vi "Read Timeout.vi"(8 "error in (no error)":errorcluster, 11 "Repeat Until Timeout in":refnum<class "bt_Repeat Until Timeout.lvclass">) -> (0 "error out":errorcluster, 2 "Timeout":dbl, 3 "Repeat Until Timeout out":refnum<class "bt_Repeat Until Timeout.lvclass">)   [LabVIEW 2021, in "BT.lvlib" / "bt_Repeat Until Timeout.lvclass"]
uses:
  bt_Repeat Until Timeout.lvclass
  bt_Repeat Until Timeout.lvclass/bt_Repeat Until Timeout.ctl
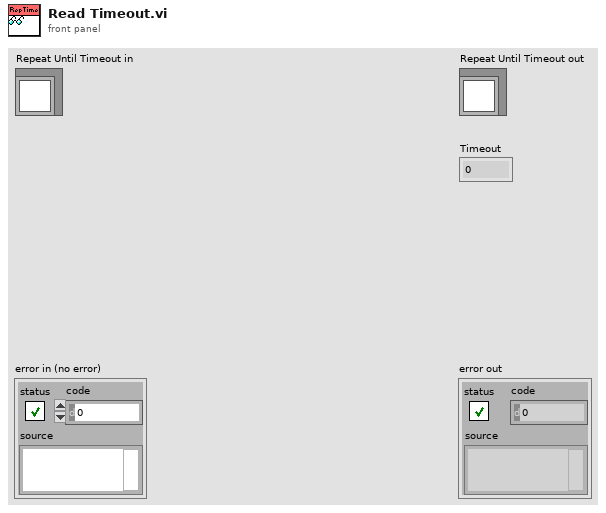
[diagram p1: front panel]
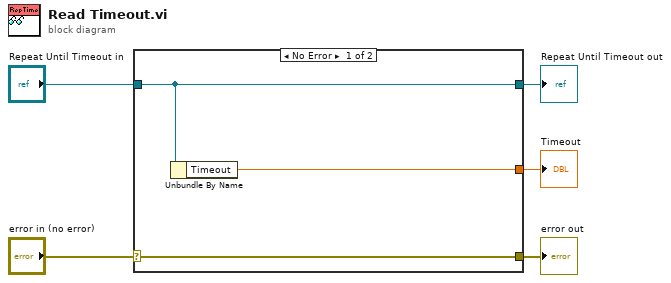
[diagram p0: block diagram]
diagram:
  n1 = case shown="No Error" "error in (no error)" {
    selector: "error in (no error)" -> [w8 w9]
    tunnel: [w8 w9] -> w4
    tunnel: [w7 w10] -> w2
    tunnel: "Repeat Until Timeout in" -> [w7 w10]
    tunnel: [w6 _] -> w1
    frame No Error {
      n2 = Unbundle By Name(w7) -> ("Timeout"=w6:dbl)
    }
    frame Error {
    }
  }
  "error out" <- w4
  "Repeat Until Timeout out" <- w2
  "Timeout" <- w1
